vi "Encoder Reset.vi"(0 "Reset Encoder Left?":bool, 1 "Left Encoder RefNum":string="My Encoder RefNum", 2 "Reset Both?":bool, 3 "Reset Encoder Right?":bool, 4 "Right Encocer Refnum":string="My Encoder RefNum") -> ()   [LabVIEW 2017]
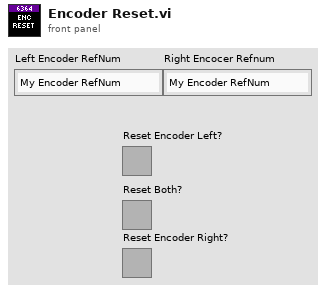
[diagram p1: front panel]
types:
  T1 = typedef "WPI_EncoderDevRef.ctl" = cluster{"DevStatus":errorcluster, "EncoderIndex":T2, "CounterIndex":T3, "DistancePerCount":dbl, "Decoding Type":T4}
  T2 = typedef "FPGA_EncoderIdx.ctl" = enum8{"Enc 0", "Enc 1", "Enc 2", "Enc 3", "Enc 4", "Enc 5", "Enc 6", "Enc 7", "Invalid"}
  T3 = typedef "FPGA_CounterCtrSystemIndex.ctl" = enum8{"Ctr 0", "Ctr 1", "Ctr 2", "Ctr 3", "Ctr 4", "Ctr 5", "Ctr 6", "Ctr 7", "Invalid"}
  T4 = typedef "WPI_EncoderType.ctl" = enum16{"1x", "2x", "4x"}
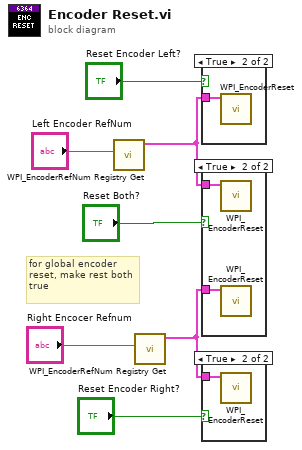
[diagram p0: block diagram]
diagram:
  # "for global encoder reset, make rest both true"
  n1 = call <vilib>:"WPI_EncoderRefNum Registry Get.vi"("refnum name"="Left Encoder RefNum") -> ("EncoderDevRef"=w4:T1)  [unwired: 9 in, 1 out]
  n2 = call <vilib>:"WPI_EncoderRefNum Registry Get.vi"("refnum name"="Right Encocer Refnum") -> ("EncoderDevRef"=w3:T1)  [unwired: 9 in, 1 out]
  n3 = case shown="True" "Reset Encoder Left?" {
    tunnel: w4 -> [_ w8]
    frame False {
    }
    frame True {
      n4 = call <vilib>:"WPI_EncoderReset.vi"("EncoderDevRef"=w8) -> ()  [unwired: 9 in, 2 out]
    }
  }
  n5 = case shown="True" "Reset Both?" {
    tunnel: w4 -> [_ w10]
    tunnel: w3 -> [_ w9]
    frame False {
    }
    frame True {
      n6 = call <vilib>:"WPI_EncoderReset.vi"("EncoderDevRef"=w10) -> ()  [unwired: 9 in, 2 out]
      n7 = call <vilib>:"WPI_EncoderReset.vi"("EncoderDevRef"=w9) -> ()  [unwired: 9 in, 2 out]
    }
  }
  n8 = case shown="True" "Reset Encoder Right?" {
    tunnel: w3 -> [_ w11]
    frame False {
    }
    frame True {
      n9 = call <vilib>:"WPI_EncoderReset.vi"("EncoderDevRef"=w11) -> ()  [unwired: 9 in, 2 out]
    }
  }
